vi "3d_weight_height.vi"() -> ()   [LabVIEW 2022 SP3]
uses:
  <vilib>/Math Plots/3D Math Plots/3D Scatter/3D Scatter XCtrl/3D Scatter.xctl
  <vilib>/Utility/file.llb/Read Delimited Spreadsheet (string).vi
  <vilib>/Math Plots/3D Math Plots/3D Scatter/3D Scatter Datatype/Public/Plot Helper (Vector).vi
  <vilib>/Math Plots/3D Math Plots/3D Scatter/3D Scatter Datatype/3D Scatter Datatype.lvclass
panel:
  out "3D Scatter":refnum<class "3D Plot Datatype.lvclass">[](xcontrol)
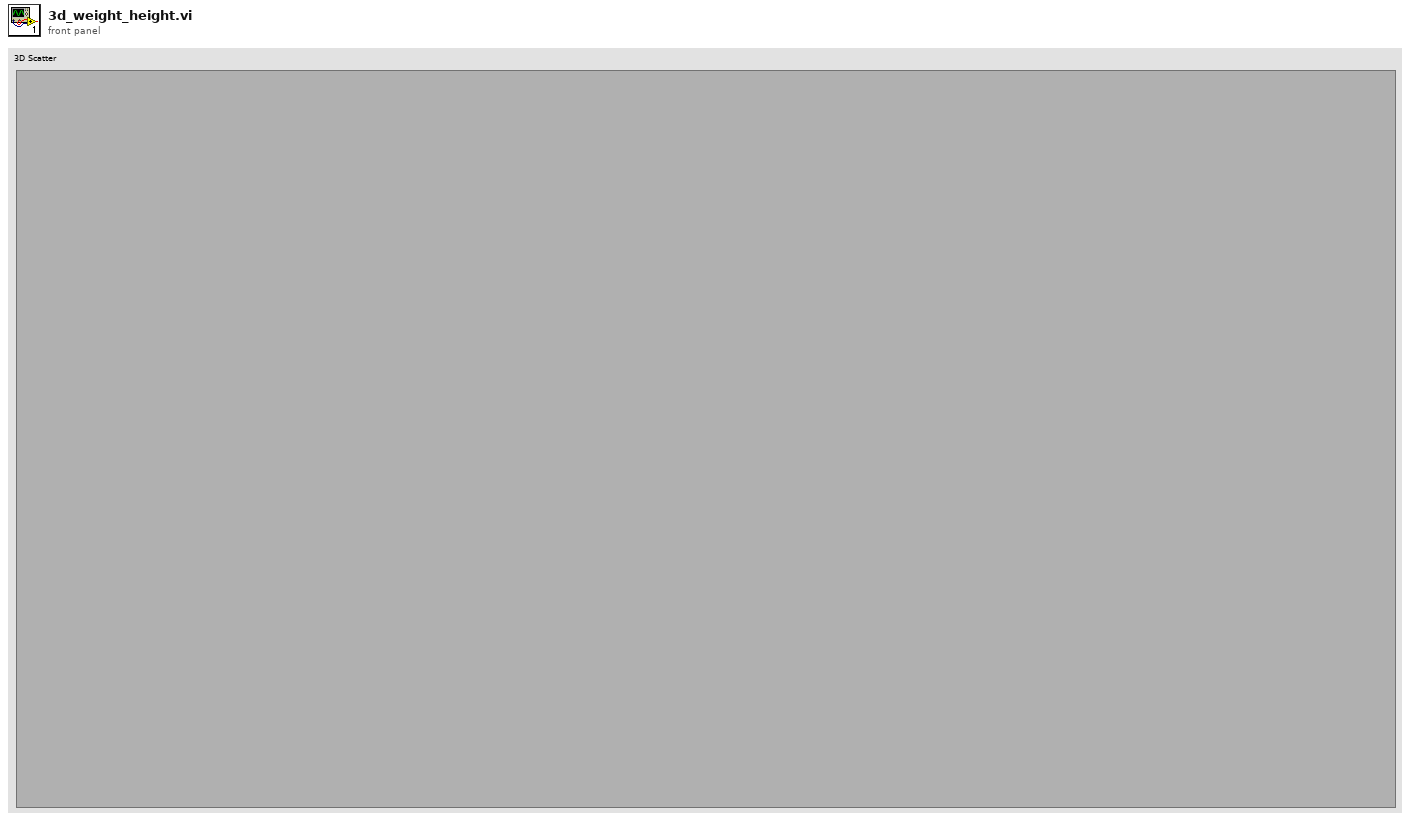
[diagram p1: front panel]
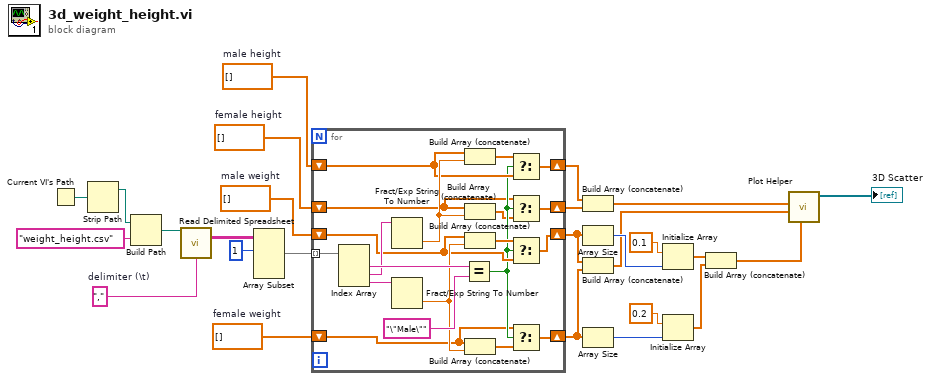
[diagram p0: block diagram]
diagram:
  w15 = dbl[] []  # female weight
  w16 = dbl[] []  # female height
  w17 = dbl[] []  # male weight
  w18 = dbl[] []  # male height
  w22 = ","  # delimiter (\t)
  n1 = Current VI's Path() -> (path=w26:path)
  n2 = Strip Path(path=w26) -> (stripped path=w25:path)  [unwired: 1 out]
  n3 = Build Path(base path=w25, name or relative path="weight_height.csv") -> (appended path=w23:path)
  n4 = call-poly <vilib>:"Read Delimited Spreadsheet.vi"("file path (dialog if empty)"=w23, "delimiter (\\t)"=w22) -> ("all rows"=w21:string[][])  [unwired: 8 in, 5 out]
  n5 = Array Subset(array=w21, index (row)=1 ("index")) -> (w19:string[][])  [unwired: 3 in]
  n6 = for {
    tunnel: w19 -> [w46] mode=indexing
    shift-right: [w41] -> w9
    shift-left: w18 -> [w35]
    shift-right: [w38] -> w6
    shift-left: w17 -> [w34]
    shift-right: [w27] -> w8
    shift-left: w16 -> [w32]
    shift-right: [w28] -> w5
    shift-left: w15 -> [w31]
    n7 = Index Array(array=w46) -> (element #1=w45:string, element #2=w43:string, element #3=w39:string)  [unwired: 3 in]
    n8 = Fract/Exp String To Number(string=w43) -> (number=w36:dbl)  [unwired: 3 in, 1 out]
    n9 = Fract/Exp String To Number(string=w39) -> (number=w37:dbl)  [unwired: 3 in, 1 out]
    n10 = Equal?(x=w45, y="\"Male\"") -> (x = y?=w33:bool)
    n11 = Build Array (concatenate)(w35, w36) -> (w42:dbl[])
    n12 = Build Array (concatenate)(w32, w36) -> (w30:dbl[])
    n13 = Build Array (concatenate)(w34, w37) -> (w40:dbl[])
    n14 = Build Array (concatenate)(w31, w37) -> (w29:dbl[])
    n15 = Select(t=w42, s=w33, f=w35) -> (s? t:f=w41:dbl[])
    n16 = Select(t=w32, s=w33, f=w30) -> (s? t:f=w27:dbl[])
    n17 = Select(t=w40, s=w33, f=w34) -> (s? t:f=w38:dbl[])
    n18 = Select(t=w31, s=w33, f=w29) -> (s? t:f=w28:dbl[])
  }
  n19 = Build Array (concatenate)(w9, w8) -> (w7:dbl[])
  n20 = Array Size(array=w6) -> (size(s)=w13:i32)
  n21 = Build Array (concatenate)(w6, w5) -> (w4:dbl[])
  n22 = Array Size(array=w5) -> (size(s)=w12:i32)
  n23 = Initialize Array(0.1 ("Data"), w13) -> (w3:dbl[])
  n24 = Initialize Array(0.2 ("Data"), w12) -> (w2:dbl[])
  n25 = Build Array (concatenate)(w3, w2) -> (w1:dbl[])
  n26 = call-poly <vilib>:"Plot Helper.vi"("z vector"=w1, "y vector"=w4, "x vector"=w7) -> ("3D Plot lvclass Array out"=→"3D Scatter":refnum<class "3D Plot Datatype.lvclass">[])  [unwired: 3 in, 5 out]
